vi "init.vi"(8 "error in (no error)":errorcluster, 11 "ForceSensor in":refnum<class "ForceSensorCalculatorTC.lvclass">) -> (0 "error out":errorcluster, 3 "ForceSensor out":refnum<class "ForceSensorCalculatorTC.lvclass">)   [LabVIEW 2015, in "ForceSensorCalculatorTC.lvclass"]
uses:
  ForceSensorCalculatorTC.lvclass
  <userlib>/Common/Devices/ForceSensorCalculator/Config/ForceSensorCalculator.ctl
  <userlib>/Common/Devices/ForceSensorCalculator/ForceSensorCalculator/ForceSensorCalculator.lvclass/ForceSensorCalculator.ctl
  <userlib>/Common/Devices/ForceSensorCalculator/ForceSensorCalculator/ForceSensorCalculator.lvclass
  <userlib>/Common/Devices/ForceSensorCalculator/ForceSensorCalculator.lvlib
  ConfigurationThisComponent/ConfigurationThisComponent.lvclass
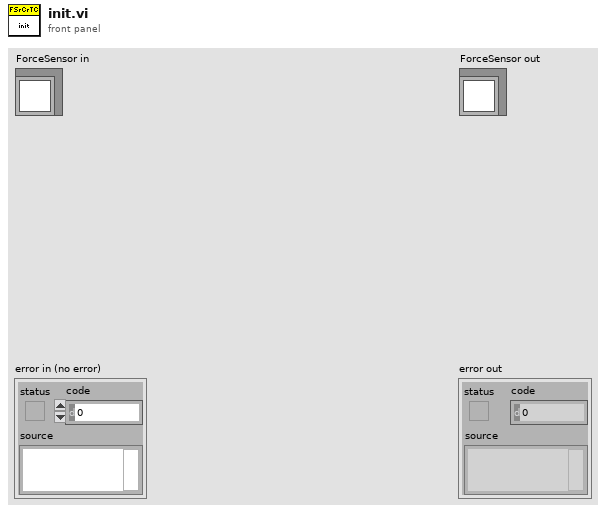
[diagram p1: front panel]
types:
  T1 = typedef "ForceSensorCalculator.lvlib/ForceSensorCalculator.ctl" = cluster{"Capacity":dbl[unit], "Sensitivity":dbl[unit]}
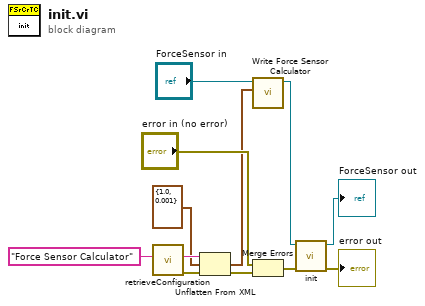
[diagram p0: block diagram]
diagram:
  n1 = call "retrieveConfiguration.vi"("configName"="Force Sensor Calculator") -> ("error out"=w9:errorcluster, "xmlConfig"=w8:string)  [unwired: 8 in, 1 out]
  n2 = Unflatten From XML(xml string=w8, type=T1 {"Capacity"=1.0, "Sensitivity"=0.001} ("Force Sensor Calculator"), error in (no error)=w9) -> (value=w2:T1, error out=w6:errorcluster)
  n3 = call <userlib>:"Write Force Sensor Calculator.vi"("Force Sensor Calculator"=w2, "ForceSensorCalculator in"="ForceSensor in") -> ("ForceSensorCalculator out"=w3:refnum<class "ForceSensorCalculatorTC.lvclass">)  [unwired: 9 in]
  n4 = Merge Errors("error in (no error)", w6) -> (w5:errorcluster)
  n5 = call-parent "init.vi"("error in (no error)"=w5, "ForceSensor in"=w3) -> ("error out"=→"error out":errorcluster, "ForceSensor out"=→"ForceSensor out":refnum<class "ForceSensorCalculatorTC.lvclass">)  [unwired: 8 in]
